vi "Timestamp info.vi"(8 "error in (no error)":errorcluster, 11 "Variant":variant) -> (0 "error out":errorcluster, 3 "child strings":string[](array[string]))   [LabVIEW 2020, in "DSF Configuration Utility.lvlib"]
uses:
  DSF Configuration Utility.lvlib
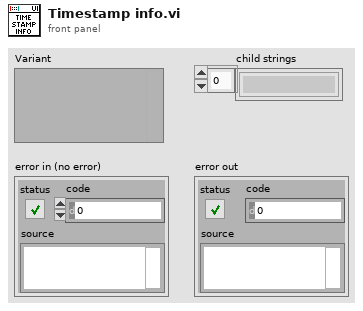
[diagram p1: front panel]
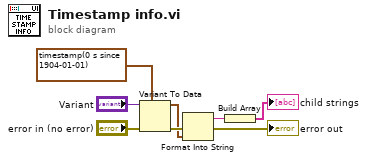
[diagram p0: block diagram]
diagram:
  n1 = Variant To Data(error in="error in (no error)", type=timestamp(0 s since 1904-01-01) ("Time Stamp"), Variant="Variant") -> (data=w3:timestamp, error out=w7:errorcluster)
  n2 = Format Into String(error in=w7, w3) -> (resulting string=w4:string, error out=→"error out":errorcluster)  [unwired: 2 in]
  n3 = Build Array(w4) -> (→"child strings":string[])
